vi "Flash Firmware.vi"(8 "error in":errorcluster, 10 "path to code":path, 11 "spark reference in":T1) -> (0 "error out":errorcluster, 3 "spark reference out":T1)   [LabVIEW 2013, in "Spark API.lvlib"]
doc: "Calls curl on the commandline to upload new firmware to the currently connected Spark device."
uses:
  Spark API.lvlib
  Controls/Spark Reference.ctl
  <vilib>/httpClient/ClientHandle.ctl
  Controls/Device Query JSON.ctl
  <vilib>/httpClient/LabVIEWHTTPClient.lvlib
panel:
  # "The LabVIEW HTTP Client doesn't support multipart/form PUTs, so we're using curl directly. If cURL isn't installed, or if this is on a non-Mac platform, this will likely generate an error"
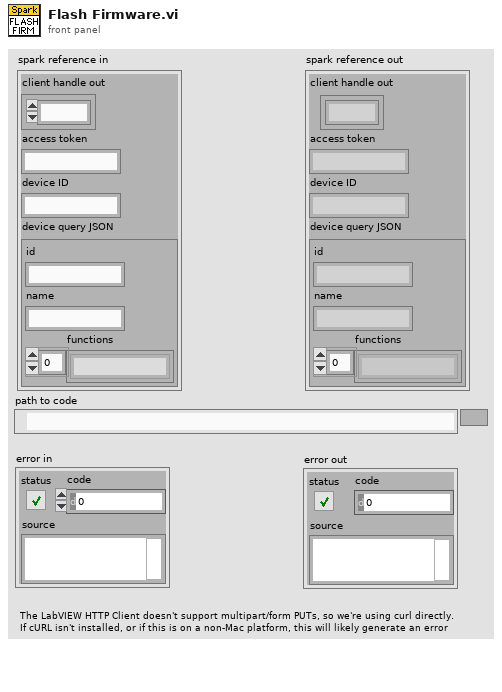
[diagram p1: front panel]
types:
  T1 = typedef "Spark API.lvlib/Spark Reference.ctl" = cluster{"client handle out":T2, "access token":string, "device ID":string, "device query JSON":T3}
  T2 = typedef "LabVIEWHTTPClient.lvlib/ClientHandle.ctl" = refnum<k1>
  T3 = typedef "Spark API.lvlib/Device Query JSON.ctl" = cluster{"id":string, "name":string, "functions":string[]}
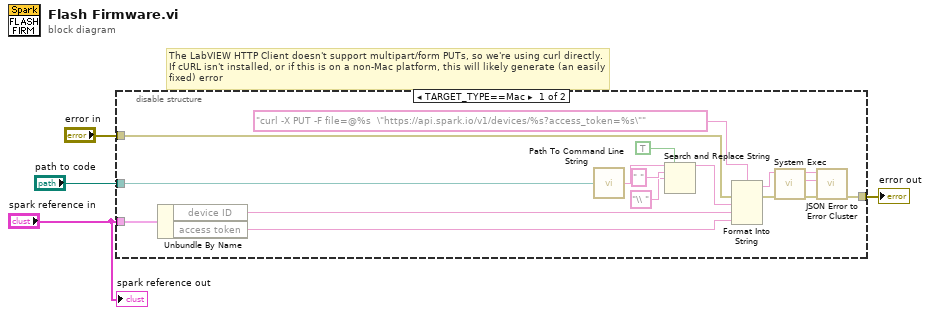
[diagram p0: block diagram]
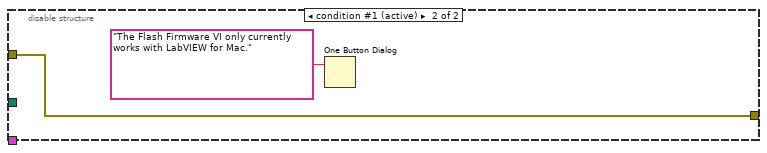
[diagram p2: hidden frame]
diagram:
  # "The LabVIEW HTTP Client doesn't support multipart/form PUTs, so we're using curl directly. If cURL isn't installed, or if this is on a non-Mac platform, this will likely generate (an easily fixed) error"
  n1 = disable-structure shown="TARGET_TYPE==Mac" {
    disable-tunnel: "error in" -> [w20 w23]
    disable-tunnel: "spark reference in" -> [w19 _]
    disable-tunnel: "path to code" -> [w17 _]
    disable-tunnel: [w5 w23] -> w1
    frame condition #0 {
      n2 = Unbundle By Name(w19) -> ("device ID"=w16:string, "access token"=w18:string)
      n3 = call <vilib>:"Path To Command Line String.vi"("path"=w17) -> ("string"=w11:string)
      n4 = Search and Replace String(replace all?=TRUE ("replace all? (F)"), input string=w11, search string=" ", replace string="\\ " ("replace string (\"\")")) -> (result string=w12:string)  [unwired: 4 in, 3 out]
      n5 = Format Into String(format string="curl -X PUT -F file=@%s  \"https://api.spark.io/v1/devices/%s?access_token=%s\"" ("url"), error in=w20, w12, w16, w18) -> (resulting string=w15:string, error out=w14:errorcluster)  [unwired: 1 in]
      n6 = call <vilib>:"System Exec.vi"("error in (no error)"=w14, "command line"=w15) -> ("error out"=w13:errorcluster, "standard error"=w7:string, "standard output"=w6:string)  [unwired: 6 in, 1 out]
      n7 = call "JSON Error to Error Cluster.vi"("error in (no error)"=w13, "headers"=w7, "JSON string"=w6) -> ("error out"=w5:errorcluster)  [unwired: 8 in]
    }
    frame condition #1 (active) {
      n8 = One Button Dialog(message="The Flash Firmware VI only currently works with LabVIEW for Mac.") -> ()  [unwired: 1 in, 1 out]
    }
  }
  "error out" <- w1
  "spark reference out" <- "spark reference in"
